vi "NT Get Topic.vi"(8 "error in (no error)":errorcluster, 11 "name":string) -> (0 "error out":errorcluster, 3 "topicHandle":u32)   [LabVIEW 2025]
uses:
  FRC_NetworkTablesLV.dll
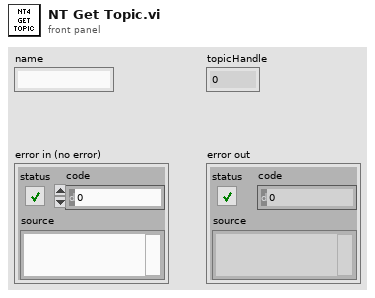
[diagram p1: front panel]
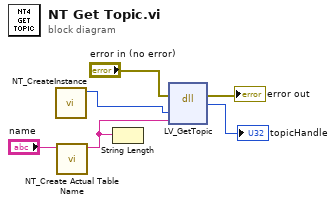
[diagram p0: block diagram]
diagram:
  n1 = call <vilib>:"NT_CreateInstance.vi"() -> ("InstanceHandle"=w4:u64)  [unwired: 10 in, 1 out]
  n2 = call <vilib>:"NT_Create Actual Table Name.vi"("Name or Path"="name") -> ("Absolute Path"=w2:string)  [unwired: 10 in]
  n3 = String Length(string=w2) -> ()  [unwired: 1 out]
  n4 = dll-call lib="FRC_NetworkTablesLV.*" fn="LV_GetTopic"(error in="error in (no error)", "InstHandle"=w4, "name"=w2) -> (error out=→"error out":errorcluster, "topicHandle"=→"topicHandle":u32)  [unwired: 4 in, 1 out]
